vi "温度曲线显示.vi"() -> ()   [LabVIEW 2016, in "斯坦道通用流路CODmn.lvlib"]
panel:
  out "显示值":string
  in  "历史曲线":bool
  in  "单选按钮":enum32{"消解温度曲线", "注射器温度曲线"}(radio)
  in  "关闭":bool
  out "波形图":sgl[](graph)
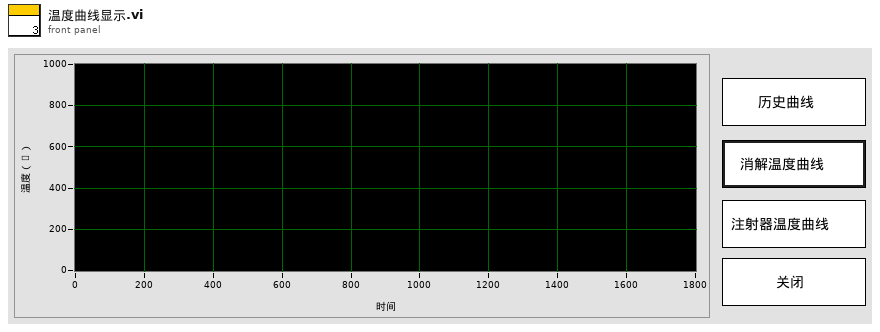
[diagram p1: front panel]
types:
  T1 = typedef "LVPoint32TypeDef.ctl" = cluster{"Horizontal":i32, "Vertical":i32}
  T2 = typedef "SingleStepTestV3.lvlib/SingleStepTestV3.lvclass/仪器版本.ctl" = enum16{"V3.1版", "V4版", "V3版", "V4.2版"}
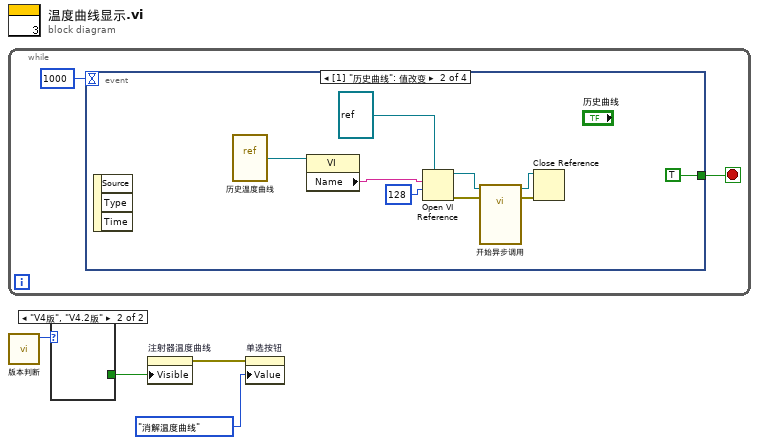
[diagram p0: block diagram]
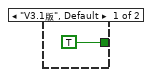
[diagram p2: hidden frame]
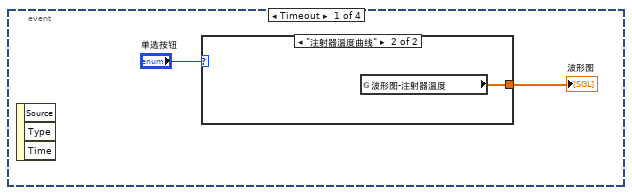
[diagram p3: hidden frame]
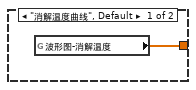
[diagram p4: hidden frame]
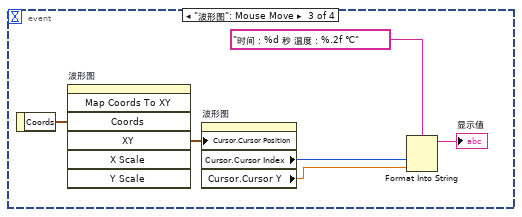
[diagram p5: hidden frame]
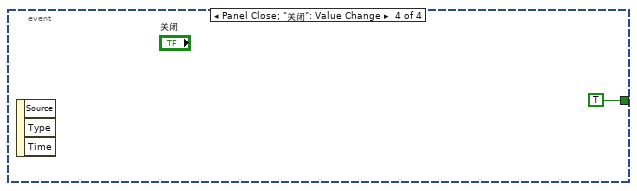
[diagram p6: hidden frame]
diagram:
  n1 = while {
    stop <- w6 stop-if-true
    n2 = event shown="[1] \"历史曲线\": 值改变" {
      selector: _ -> [_ _ _ _]
      dyn-events: _ -> [_ _ _ _]
      timeout: 1000 -> [_ _ _ _]
      tunnel: [_ TRUE _ TRUE] -> w6
      event Timeout {
        n3 = event-data() -> ()  [unwired: 1 in, 3 out]
        n4 = case shown="\"注射器温度曲线\"" "单选按钮" {
          tunnel: [w9 w10] -> w7
          frame "消解温度曲线", Default {
            n5 = global read "VAR总磷总氮全局变量.vi" "波形图-消解温度"() -> (w9:sgl[])
          }
          frame "注射器温度曲线" {
            n6 = global read "VAR总磷总氮全局变量.vi" "波形图-注射器温度"() -> (w10:sgl[])
          }
        }
        "波形图" <- w7
      }
      event "历史曲线": Value Change {
        n7 = event-data() -> ()  [unwired: 1 in, 3 out]
        n8 = vi-ref "历史温度曲线.vi"() -> (w11:refnum<vi>)
        n9 = property class="VI"(reference=w11) -> ("Name"=w12:string)  [unwired: 1 in, 2 out]
        n10 = Open VI Reference(type specifier VI Refnum (for type only)=refnum<vi> refnum, vi path=w12, options=128 ("选项")) -> (vi reference=w15:refnum<vi>, error out=w16:errorcluster)  [unwired: 3 in]
        n11 = call-by-ref "开始异步调用"(reference=w15, error in=w16) -> (reference out=w17:refnum<vi>, error out=w18:errorcluster)  [unwired: 12 in]
        n12 = Close Reference(reference=w17, error in (no error)=w18) -> ()  [unwired: 1 out]
      }
      event "波形图": Mouse Move {
        n13 = event-data() -> ("Coords"=w25:T1)  [unwired: 1 in]
        n14 = invoke on="波形图" class="WFGraph (严格)" method="Map Coords To XY"("Coords"=w25) -> ("XY"=w24:cluster{"X":dbl, "Y":dbl})  [unwired: 6 in, 6 out]
        n15 = property on="波形图" class="WFGraph (严格)"("Cursor.Cursor Position"=w24) -> ("Cursor.Cursor Index"=w21:i32, "Cursor.Cursor Y"=w20:dbl)  [unwired: 2 in, 2 out]
        n16 = Format Into String(format string="时间：%d 秒 温度：%.2f ℃" ("格式字符串"), w21, w20) -> (resulting string=→"显示值":string)  [unwired: 2 in, 1 out]
      }
      event Panel Close; "关闭": Value Change {
        n17 = event-data() -> ()  [unwired: 1 in, 3 out]
      }
    }
  }
  n18 = call "版本判断.vi"() -> ("仪器版本"=w4:T2)  [unwired: 11 in]
  n19 = case shown="\"V4版\", \"V4.2版\"" w4 {
    tunnel: [TRUE _] -> w3
    frame "V3.1版", Default {
    }
    frame "V4版", "V4.2版" {
    }
  }
  n20 = property on="注射器温度曲线" class="Bool (严格)"("Visible"=w3) -> (error out=w1:errorcluster)  [unwired: 2 in, 1 out]
  n21 = property on="单选按钮" class="RadioBtnsControl (严格)"(error in=w1, "Value"=enum32{"消解温度曲线", "注射器温度曲线"}."消解温度曲线" ("单选按钮")) -> ()  [unwired: 1 in, 2 out]
